vi "Dashboard Main.vi"() -> ()   [LabVIEW 2018]
uses:
  <vilib>/Utility/miscctls.llb/LVRowAndColumnTypeDef.ctl
  <vilib>/event_ctls.llb/eventvkey.ctl
  <vilib>/Rock Robotics/Network Tables/NT Read Boolean Array.vi
  <vilib>/Rock Robotics/Network Tables/NT Read Numeric Array.vi
  <vilib>/Rock Robotics/Network Tables/NT Write Numeric Array.vi
  <vilib>/Rock Robotics/Network Tables/NT Write String Array.vi
  <vilib>/Rock Robotics/WPI/Dashboard/WPI_DashboardLogging Global.vi
panel:
  in  "Camera Name":string(combo)="No Camera Selection"
  in  "Camera Settings Right":T1={"Frame Rate"=30, "Compression"=30, "Size"=1, "DB Camera Config"=FALSE} {"Frame Rate" scale=1.0..30.0; "Compression" scale=100.0..-1.0; "Size" items=["640x480", "320x240", "160x120"]}
  in  "Camera Name Right":string(combo)="No Camera Selection"
  out "Camera Perf":string
  in  "Camera Settings":T1={"Frame Rate"=30, "Compression"=30, "Size"=1, "DB Camera Config"=FALSE} {"Frame Rate" scale=1.0..30.0; "Compression" scale=100.0..-1.0; "Size" items=["640x480", "320x240", "160x120"]}
  in  "TCP":refnum<k5>
  in  "Rec Mode":enum32{"Stop", "Record", "Playback"}(radio)
  out "Robot IP":string
  out "Image Message":string="Timeout in Camera Communications"
  in  "Dashboard Tab":T2(tab)
  out "Error Message:":string
  in  "Run Automated:":bool
  out "NT Connection":bool
  out "Mode":T3(ring)=enum."Auto Disabled"
  out "Right Camera Perf":cluster{"Bandwidth (Mbps)":dbl, "FPS":dbl}
  out "Front Left Setpoint:":dbl(knob)
  out "Front Right Setpoint:":dbl(knob)
  out "Back Left Setpoint:":dbl(knob)
  out "Back Right Setpoint:":dbl(knob)
  out "Reversed Modules":bool[](array[boolean])
  in  "Write Swerve Offsets:":bool
  in  "Task:":string(combo)
  out "PositionIndicator":bool
  out "TaskIndicator":bool
  in  "Start Position:":string(combo)
  out "Camera Image Right":T4(plugin-control)
  in  "CheckList":i32(listbox)
  in  "Test Slider":dbl(slide) scale=0.0..100.0 scale format="%#_3g"
  in  "On/Off":bool caption="Solenoid"
  in  "Test Name":u16(ring) items=["Select the test to run..."]
  in  "Test Tree":string(tree)
  in  "Motor":cluster{"Value":dbl, "Enable":bool} {"Value" scale=-1.0..1.0 scale format="%#_3g"}
  out "Progress":T5 {"Test Progress" scale=0.0..100.0}
  in  "Rev/Fwd":cluster{"Forward":bool, "Reverse":bool}
  in  "Test Ring":u16(ring) items=["Monochrome", "Color"]
  out "Cmd Status":string
  in  "Execute Command":bool
  in  "Command Params":string[][](table)
  in  "Command Selection":i32(listbox)
  out "Tree":string(tree)
  out "Camera Image":T4(plugin-control)
  out "Background":bool
  # "HW"
  # "HW"
  # "Swerve Modules:"
  # "Sandstorm Options:"
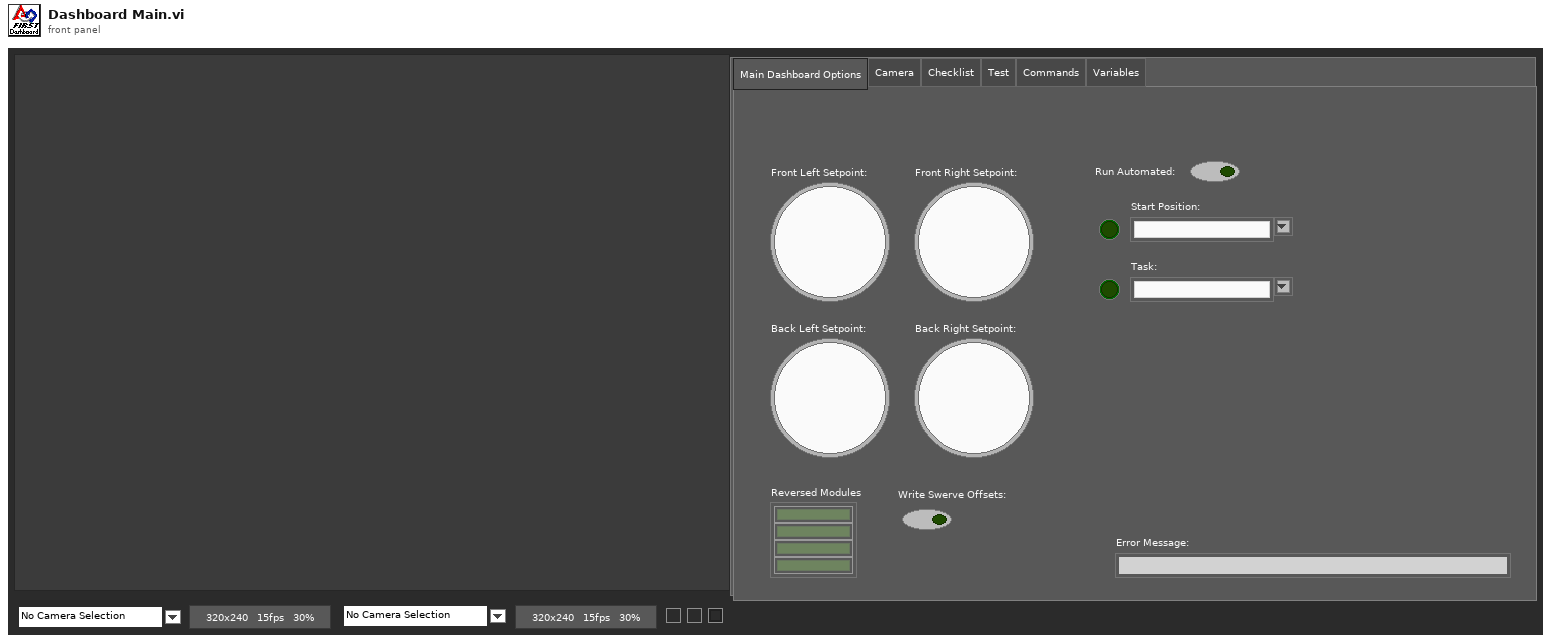
[diagram p1: front panel]
types:
  T1 = cluster{"Frame Rate":i32, "Compression":i32, "Size":u16, "DB Camera Config":bool}
  T2 = enum32{"Main Dashboard Options", "Camera", "Checklist", "Test", "Commands", "Variables"}
  T3 = enum8{"Tele-Op Disabled", "Tele-Op Enabled", "Auto Disabled", "Auto Enabled", "Test Disabled", "Test Enabled", "Disconnected", "No Code", "E-Stop"}
  T4 = typedef "IMAQ Image.ctl" = refnum<image>
  T5 = cluster{"Test Progress":u8, "Test Progress Text":string}
  T6 = cluster{"Save Path":path, "Interval (s)":dbl, "Keep":i32}
  T7 = enum32{"Drive", "Camera", "Basic", "Custom", "Test", "Commands", "Checklist", "Variables"}
  T8 = typedef "Image Type" = u32
  T9 = cluster{"IDs":cluster{"RPC field ID":u16, "Unique ID":u16}, "String":string}
  T10 = enum16{"open", "replace", "create", "open or create", "replace or create", "replace or create with confirmation"}
  T11 = cluster{"Error Strings":string, "Disable Counts":cluster{u16, u16}, "Rail Faults":cluster{u16, u16, u16}, "Robot IP":string, "DB Mode":u8, "Event Info":cluster{"Name":string, "Type":u8, "Number":u16, "Replay":u8}}
  T12 = cluster{"Storage":cluster{"Disk Free":u64, "RAM Block":u32, "RAM free":u32}, "CPU Utilization":cluster{"CPU % ISR":sgl, "CPU % Time Crit":sgl, "CPU % Timed Str":sgl, "CPU % High":sgl, "CPU % Above":sgl, "CPU % Normal":sgl, "CPU % Low":sgl}, "CAN":cluster{"% Bus Utilization":sgl, "Bus Off Cnt":u32, "TX_FIFO Full Cnt":u32, "Receive Error Cnt":u8, "Transmit Error Cnt":u8}, "HID":cluster{"HID Outputs":u32, "Rumble Low":u16, "Rumble High":u16}[]}
  T13 = cluster{"Status bits":cluster{"Test Mode":bool, "Autonomous":bool, "Enabled":bool, "Code Start":bool, "Brownout":bool, "Reserved 2":bool, "Reserved 3":bool, "E-Stop":bool}, "Code Trace":cluster{"Disabled":bool, "TeleOp":bool, "Auto":bool, "Test":bool}, "Controller Type":enum16{"unknown", "cRIO", "roboRio"}, "Code?":enum16{"unknown", "noCode", "code"}, "Battery V":dbl}
  T14 = cluster{"Control Bits":cluster{"TestMode":bool, "Autonomous":bool, "Enabled":bool, "FMS Present":bool, bool, bool, bool, "E-Stop":bool}, "Team Station ":u8, "Countdown":sgl, "Joystick Values":cluster{"Axes":dbl[], "Buttons":bool[], "POVs":i16[]}[]}
  T15 = cluster{"Camera Image":refnum<vi>, "Dashboard Tab":refnum<vi>, "Background":refnum<vi>, "Rec Mode":refnum<vi>, "Test Slider":refnum<vi>, "On/Off ":refnum<vi>, "Test Ring":refnum<vi>, "Rev/Fwd":refnum<vi>, "Test Name":refnum<vi>, "Motor":refnum<vi>, "Progress":refnum<vi>, "CheckList":refnum<vi>, "Tree":refnum<vi>, "Test Tree":refnum<vi>, "Command Params":refnum<vi>, "Command Selection":refnum<vi>, "Execute Command":refnum<vi>, "Cmd Status":refnum<vi>, "Camera Settings":refnum<vi>, "Camera Name":refnum<vi>, "Camera Perf":refnum<vi>, "Camera Settings Right":refnum<vi>, "Camera Name Right":refnum<vi>, "Camera Image Right":refnum<vi>}
  T16 = cluster{"Global Rectangle":i32[], "Contours":cluster{"Contour Type":u32, "ROI Type":u32, "Points":i32[]}[]}
  T17 = cluster{"Camera Name":string, string, "Saved DB Images Info":cluster{"Save Path":path, "Interval (s)":dbl, "Keep":i32}}
  T18 = cluster{"Camera Name Right":string, string, "Saved DB Images Info":cluster{"Save Path":path, "Interval (s)":dbl, "Keep":i32}}
  T19 = cluster{"Operation":enum16{"Update", "Clear"}, "Color Box":u32}[]
  T20 = typedef "eventvkey.ctl" = enum16{"ASCII", "Enter", "Return", "Shift", "Ctrl", "Alt", "Cmd", "Opt", "Caps", "NumLock", "Clear", "Break", "Up", "Down", "Left", "Right", "Insert", "Delete", "Home", "End", "PageUp", "PageDown", "Escape", "Help", "Pause", "ScrollLock", "F1", "F2", "F3", "F4", "F5", "F6", "F7", "F8", "F9", "F10", "F11", "F12", "F13", "F14", "F15", "F16", "F17", "F18", "F19", "F20", "F21", "F22", "F23", "F24", "Play", "VolumeUp", "VolumeDown", "Mute", "Two Byte Char"}
  T21 = cluster{"Image Size":bool, "Image Type":bool, "Pixel Value":bool, "ROI Information":bool, "Zoom Factor":bool}
  T22 = cluster{"Operation":enum16{"Update", "Clear"}, "Color Box":u32}
  T23 = typedef "LVRowAndColumnTypeDef.ctl" = cluster{"Row":i32, "Column":i32}
  T24 = cluster{"Shift":bool, "Ctrl":bool, "Alt":bool, "Cmd":bool, "Opt":bool}
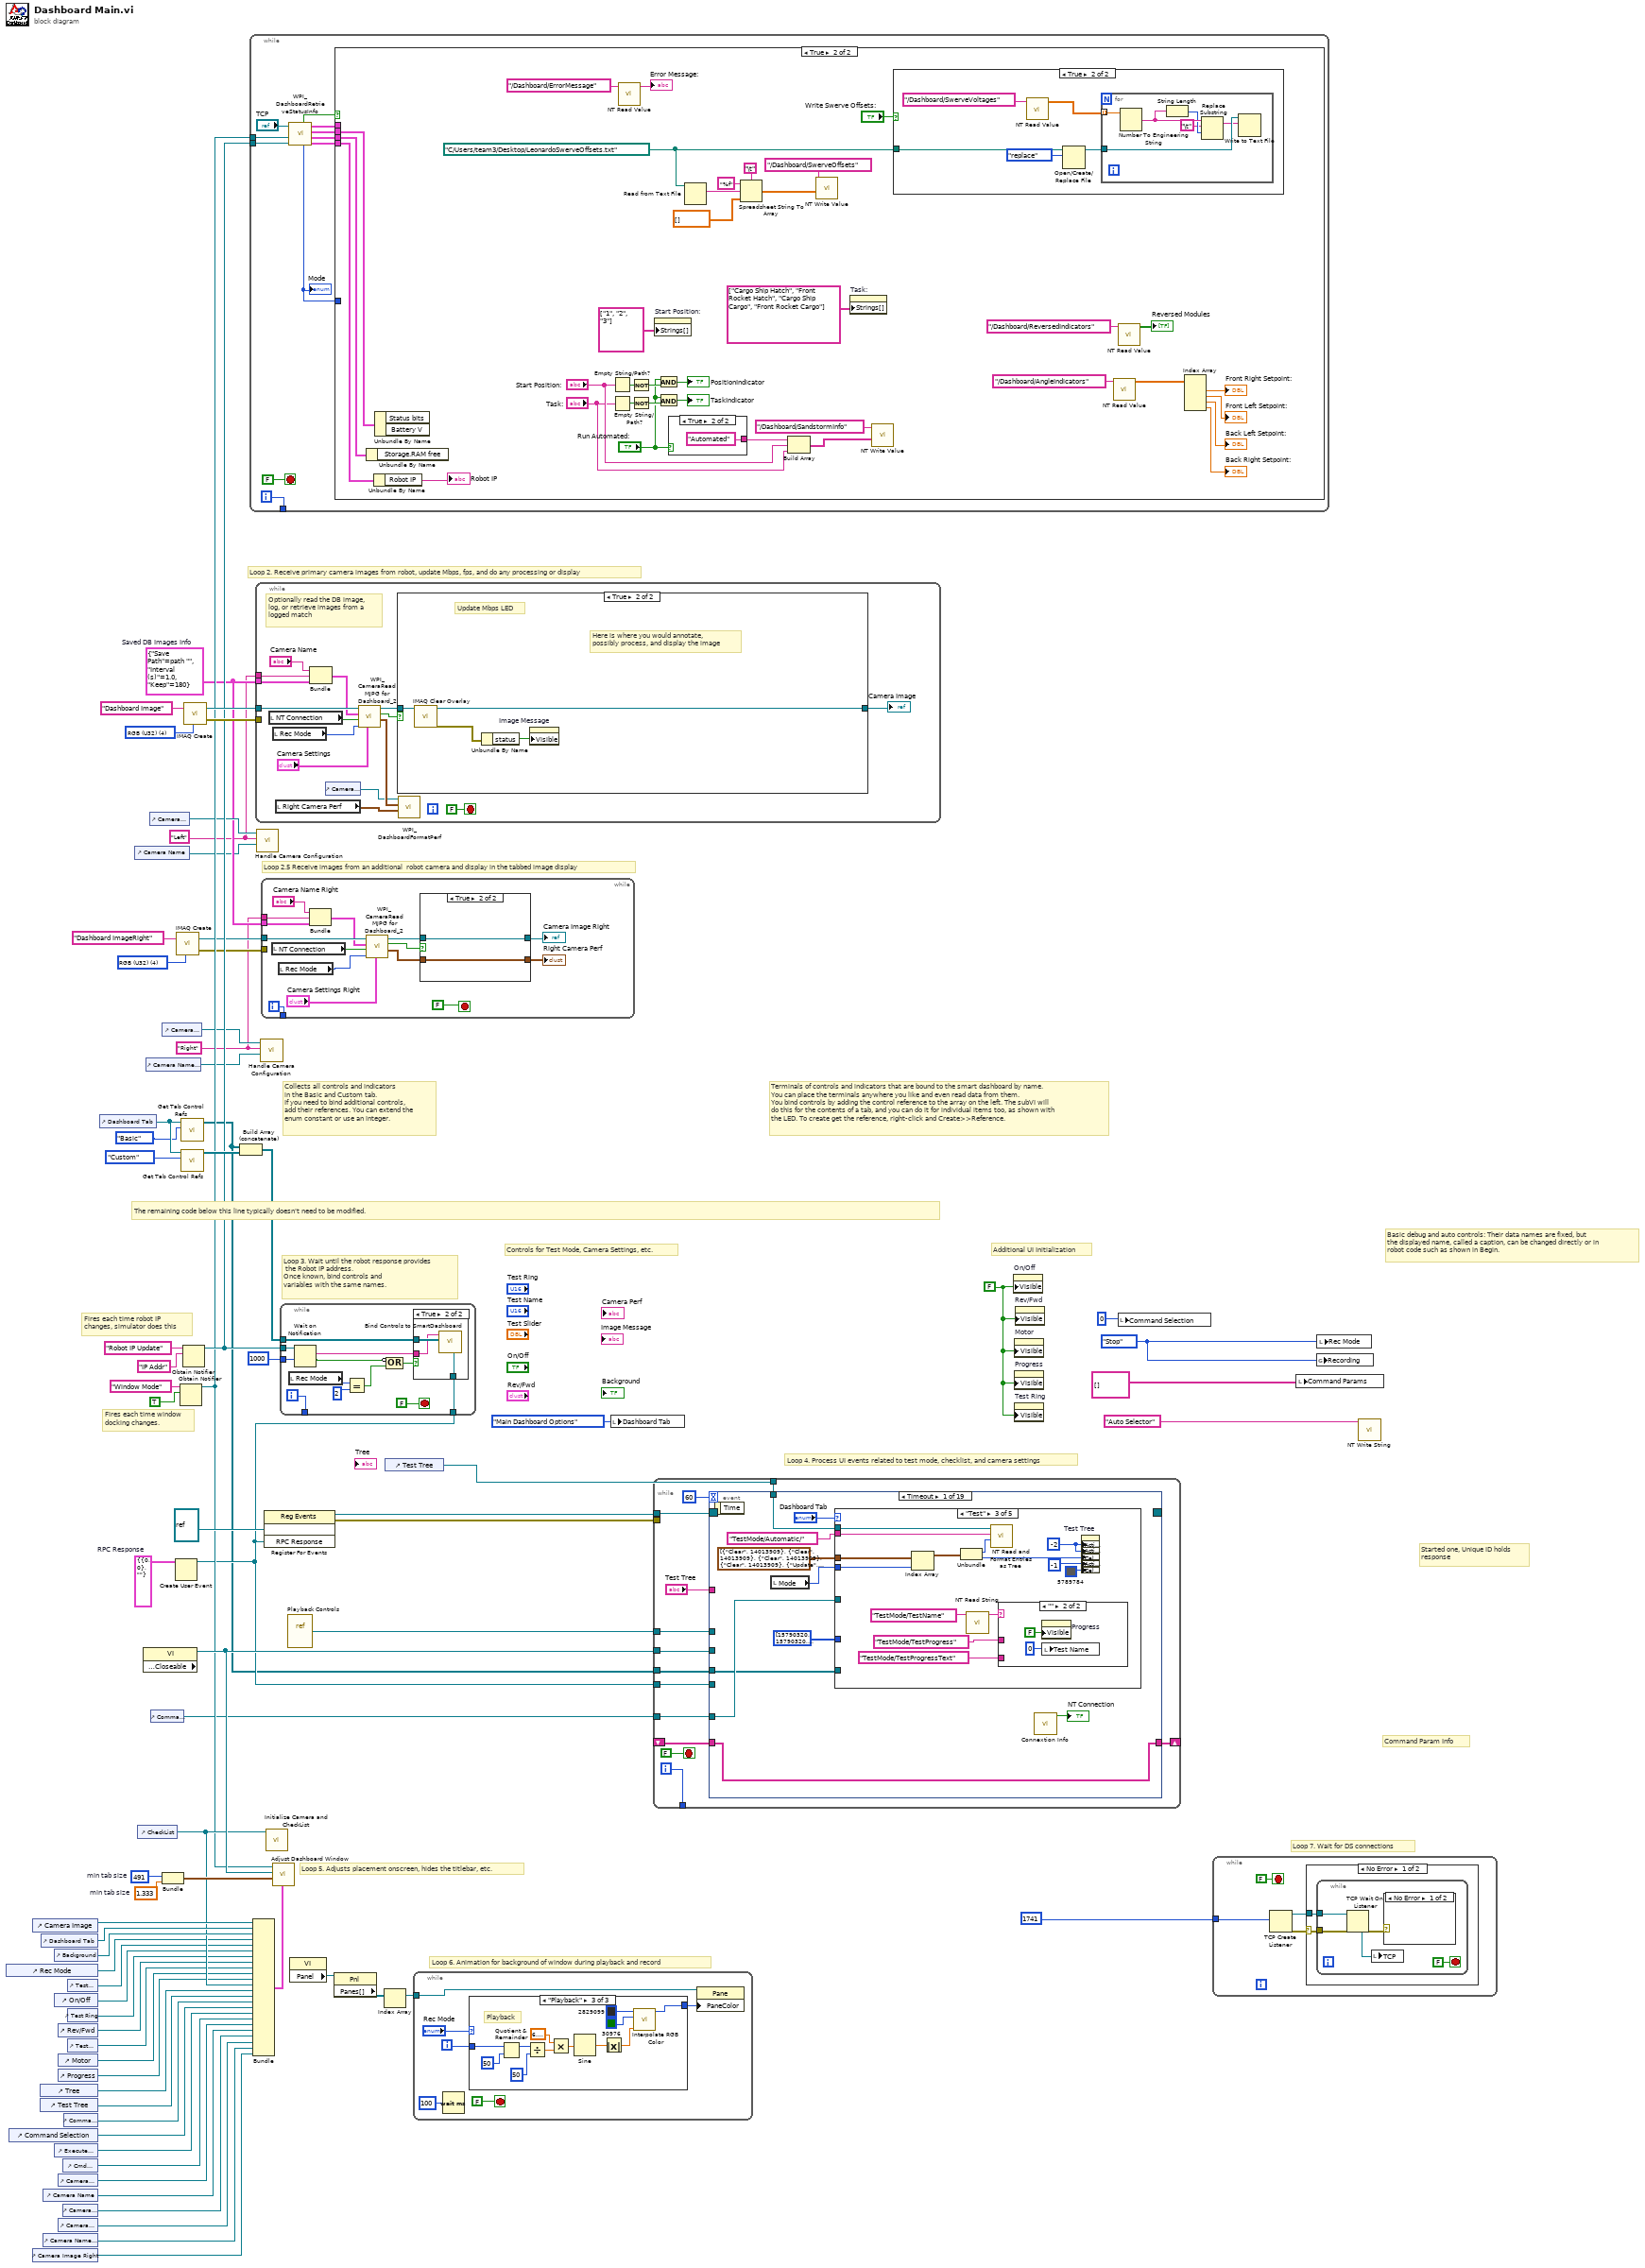
[diagram p0: block diagram]
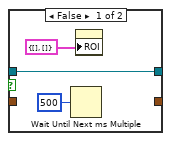
[diagram p2: hidden frame]
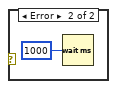
[diagram p3: hidden frame]
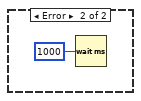
[diagram p4: hidden frame]
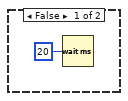
[diagram p5: hidden frame]
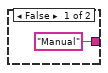
[diagram p6: hidden frame]
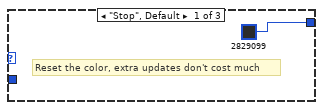
[diagram p8: hidden frame]
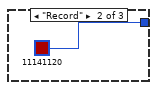
[diagram p9: hidden frame]
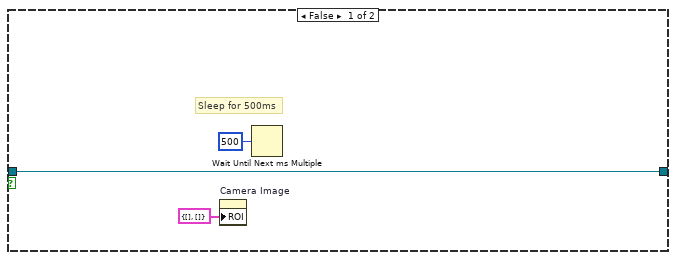
[diagram p11: hidden frame]
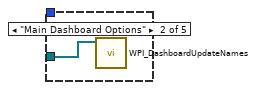
[diagram p13: hidden frame]
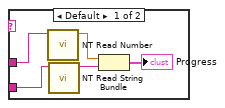
[diagram p14: hidden frame]
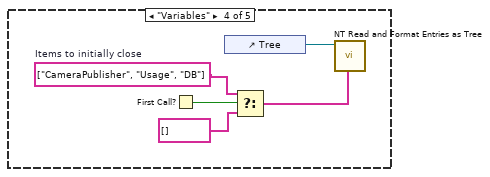
[diagram p15: hidden frame]
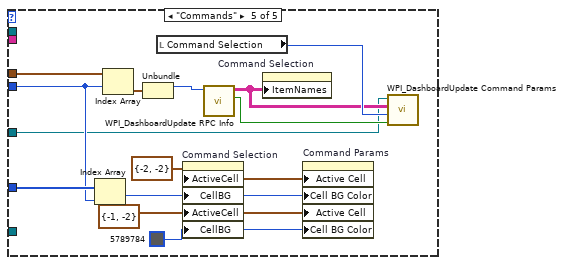
[diagram p16: hidden frame]
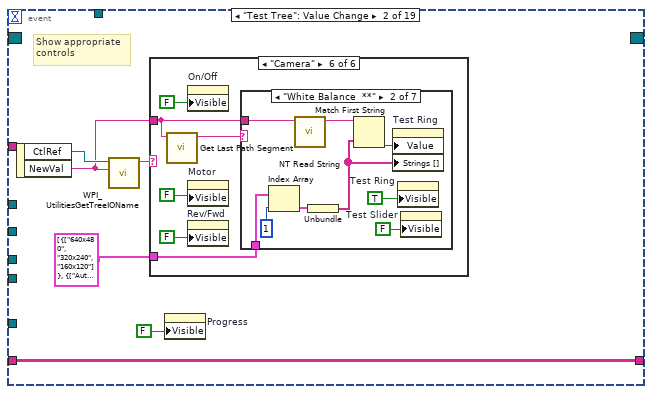
[diagram p17: hidden frame]
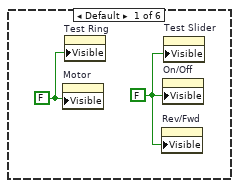
[diagram p18: hidden frame]
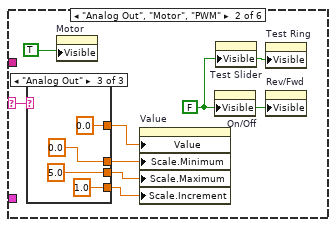
[diagram p19: hidden frame]
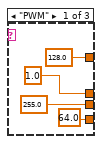
[diagram p20: hidden frame]
diagram:
  w6 = T6 {"Save Path"=path "", "Interval (s)"=1.0, "Keep"=180}  # Saved DB Images Info
  w5 = "Right"
  w4 = "Left"
  w16 = T8 4 items=["Grayscale (U8)", "Grayscale (I16)", "Grayscale (SGL)", "Complex (CSG)", "RGB (U32)", "HSL (U32)", "RGB (U64)"] ("Image Type")
  w29 = T9 {"IDs"={"RPC field ID"=0, "Unique ID"=0}, "String"=""}  # RPC Response
  w51 = 491  # min tab size
  w50 = 1.333  # min tab size
  w58 = enum32{"Stop", "Record", "Playback"}."Stop" ("Rec Mode")
  w35 = FALSE ("Visible")
  w75 = T8 4 items=["Grayscale (U8)", "Grayscale (I16)", "Grayscale (SGL)", "Complex (CSG)", "RGB (U32)", "HSL (U32)", "RGB (U64)"] ("Image Type")
  # "Loop 2.5 Receive images from an additional  robot camera and display in the tabbed image display"
  # "Command Param Info"
  # "Started one, Unique ID holds\nresponse"
  # "Loop 7. Wait for DS connections"
  # "Basic debug and auto controls: Their data names are fixed, but\nthe displayed name, called a caption, can be changed directly or in\nrobot code such as shown in Begin."
  # "Controls for Test Mode, Camera Settings, etc."
  # "Additional UI Initialization"
  # "Loop 6. Animation for background of window during playback and record"
  # "Fires each time robot IP\nchanges, simulator does this"
  # "Fires each time window\ndocking changes."
  # "Collects all controls and indicators\nin the Basic and Custom tab.\nIf you need to bind additional controls,\nadd their references. You can extend the\nenum constant or use an integer."
  # "The remaining code below this line typically doesn't need to be modified."
  # "Loop 4. Process UI events related to test mode, checklist, and camera settings"
  # "Terminals of controls and indicators that are bound to the smart dashboard by name.\nYou can place the terminals anywhere you like and even read data from them.\nYou bind controls by adding the control reference to the array on the left. The subVI will\ndo this for the contents of a tab, and you can do it for individual items too, as shown with\nthe LED. To create get the reference, right-click and Create>>Reference."
  # "Loop 3. Wait until the robot response provides\n the Robot IP address.\nOnce known, bind controls and\nvariables with the same names."
  # "Loop 5. Adjusts placement onscreen, hides the titlebar, etc."
  # "Loop 2. Receive primary camera images from robot, update Mbps, fps, and do any processing or display"
  n1 = control-ref of="Rec Mode"() -> (w41:refnum<vi>)
  n2 = control-ref of="Command Selection"() -> (w28:refnum<vi>)
  n3 = control-ref of="Camera Image"() -> (w53:refnum<vi>)
  n4 = control-ref of="Camera Image Right"() -> (w9:refnum<vi>)
  n5 = control-ref of="Tree"() -> (w45:refnum<vi>)
  n6 = control-ref of="Test Tree"() -> (w44:refnum<vi>)
  n7 = control-ref of="Dashboard Tab"() -> (w52:refnum<vi>)
  n8 = control-ref of="Camera Name"() -> (w2:refnum<vi>)
  n9 = control-ref of="Camera Name Right"() -> (w10:refnum<vi>)
  n10 = control-ref of="Background"() -> (w48:refnum<vi>)
  n11 = control-ref of="On/Off"() -> (w39:refnum<vi>)
  n12 = control-ref of="Execute Command"() -> (w30:refnum<vi>)
  n13 = control-ref of="Rev/Fwd"() -> (w37:refnum<vi>)
  n14 = control-ref of="Motor"() -> (w42:refnum<vi>)
  n15 = control-ref of="Progress"() -> (w36:refnum<vi>)
  n16 = control-ref of="Camera Settings"() -> (w21:refnum<vi>)
  n17 = control-ref of="Camera Settings Right"() -> (w11:refnum<vi>)
  n18 = control-ref of="Cmd Status"() -> (w24:refnum<vi>)
  n19 = control-ref of="Camera Perf"() -> (w20:refnum<vi>)
  n20 = control-ref of="Command Params"() -> (w31:refnum<vi>)
  n21 = control-ref of="Test Slider"() -> (w40:refnum<vi>)
  n22 = control-ref of="Test Ring"() -> (w38:refnum<vi>)
  n23 = control-ref of="Test Name"() -> (w43:refnum<vi>)
  n24 = control-ref of="Dashboard Tab"() -> (w56:refnum<vi>)
  n25 = control-ref of="Camera Name"() -> (w3:refnum<vi>)
  n26 = control-ref of="CheckList"() -> (w46:refnum<vi>)
  n27 = property class="VI" props=["Front Panel.Closeable"]() -> (reference out=w57:refnum<vi>)  [unwired: 2 in, 2 out]
  n28 = control-ref of="Camera Name Right"() -> (w12:refnum<vi>)
  n29 = control-ref of="Camera Settings"() -> (w22:refnum<vi>)
  n30 = control-ref of="Command Params"() -> (w23:refnum<vi>)
  n31 = control-ref of="Camera Settings Right"() -> (w13:refnum<vi>)
  n32 = Bundle("min tab size"=w51, "min tab size"=w50) -> (w49:cluster{"min tab size":i32, "min tab size":dbl})  [unwired: 1 in]
  n33 = Create User Event(user event datatype=w29) -> (user event=w25:refnum<user-event>)  [unwired: 1 in, 1 out]
  n34 = call "IMAQ Create"("Image Name"="Dashboard ImageRight", "Image Type"=w16) -> ("New Image"=w15:T4, "error out"=w14:errorcluster)  [unwired: 2 in, 1 out]
  n35 = Obtain Notifier(name (unnamed)="Window Mode", notification data type=TRUE) -> (notifier out=w33:refnum<notifier>)  [unwired: 2 in, 2 out]
  n36 = call <vilib>:"Get Tab Control Refs.vi"("Page Index"=T7."Basic" ("Dashboard Tab"), "TabControl in"=w56) -> ("ControlsOnPage"=w19:refnum<vi>[])  [unwired: 9 in]
  n37 = call <vilib>:"Get Tab Control Refs.vi"("Page Index"=T7."Custom" ("Dashboard Tab"), "TabControl in"=w56) -> ("ControlsOnPage"=w55:refnum<vi>[])  [unwired: 9 in]
  n38 = Obtain Notifier(name (unnamed)="Robot IP Update", notification data type="IP Addr" ("name (unnamed)")) -> (notifier out=w34:refnum<notifier>)  [unwired: 2 in, 2 out]
  n39 = call "IMAQ Create"("Image Name"="Dashboard Image", "Image Type"=w75) -> ("New Image"=w73:T4, "error out"=w72:errorcluster)  [unwired: 2 in, 1 out]
  n40 = Build Array (concatenate)(w19, w55) -> (w54:refnum<vi>[])
  n41 = while {
    tunnel: [w85] -> _
    tunnel: w34 -> [w79]
    tunnel: w33 -> [w76]
    i -> [w85]
    stop <- FALSE stop-if-true
    n42 = call <vilib>:"WPI_DashboardRetrieveStatusInfo.vi"("Binding Refnum"=w79, "Window Mode Notifier"=w76, "TCP Cnx"="TCP") -> ("Power and Errors"=w80:T11, "Robot Metrics"=w83:T12, "Status Info"=w84:T13, "Control Info"=w81:T14, "Robot Mode"=w78:T3, "Process?"=w82:bool)  [unwired: 3 in]
    "Mode" <- w78
    n43 = case shown="True" w82 {
      tunnel: w84 -> [_ w123]
      tunnel: w83 -> [_ w122]
      tunnel: w81 -> [_ _]
      tunnel: w80 -> [_ w121]
      tunnel: w78 -> [_ _]
      frame False {
        n44 = Wait (ms)(milliseconds to wait=u32 20) -> ()  [unwired: 1 out]
      }
      frame True {
        w103 = path "C:/Users/team3/Desktop/LeonardoSwerveOffsets.txt" ("file (use dialog)")
        n45 = Unbundle By Name(w122) -> ()  [unwired: 1 out]
        n46 = Unbundle By Name(w121) -> ("Robot IP"=→"Robot IP":string)
        n47 = Unbundle By Name(w123) -> ()  [unwired: 2 out]
        n48 = Empty String/Path?(string/path="Start Position:") -> (empty?=w99:bool)
        n49 = Empty String/Path?(string/path="Task:") -> (empty?=w96:bool)
        n50 = call-poly <vilib>:"NT Read Value.vi"("Name"="/Dashboard/ErrorMessage") -> ("String"=→"Error Message:":string)  [unwired: 9 in, 1 out]
        n51 = Not(x=w99) -> (.not. x?=w98:bool)
        n52 = Not(x=w96) -> (.not. x?=w97:bool)
        n53 = property on="Start Position:" class="CmbBox"("Strings[]"=string[] ["1", "2", "3"]) -> ()  [unwired: 2 in, 2 out]
        n54 = And(x="Run Automated:", y=w98) -> (x .and. y?=→"PositionIndicator":bool)
        n55 = And(x="Run Automated:", y=w97) -> (x .and. y?=→"TaskIndicator":bool)
        n56 = case shown="True" "Run Automated:" {
          tunnel: ["Manual" "Automated"] -> w93
          frame False {
          }
          frame True {
          }
        }
        n57 = Read from Text File(file (use dialog)=w103) -> (text=w117:string)  [unwired: 3 in, 3 out]
        n58 = Spreadsheet String To Array(delimiter (Tab)="\t", format string="%f", spreadsheet string=w117, array type (2D Dbl)=dbl[] []) -> (array=w116:dbl[])
        n59 = Build Array(w93, "Start Position:", "Task:") -> (w100:string[])
        n60 = call-poly <vilib>:"NT Write Value.vi"("Numeric Array"=w116, "Name"="/Dashboard/SwerveOffsets") -> ()  [unwired: 9 in, 1 out]
        n61 = property on="Task:" class="CmbBox"("Strings[]"=string[] ["Cargo Ship Hatch", "Front Rocket Hatch", "Cargo Ship Cargo", "Front Rocket Cargo"]) -> ()  [unwired: 2 in, 2 out]
        n62 = call-poly <vilib>:"NT Write Value.vi"("String Array"=w100, "Name"="/Dashboard/SandstormInfo") -> ()  [unwired: 9 in, 1 out]
        n63 = case shown="True" "Write Swerve Offsets:" {
          tunnel: w103 -> [_ w127]
          frame False {
          }
          frame True {
            n64 = call-poly <vilib>:"NT Read Value.vi"("Name"="/Dashboard/SwerveVoltages") -> ("Numeric Array"=w126:dbl[])  [unwired: 9 in, 1 out]
            n65 = Open/Create/Replace File(file path (use dialog)=w127, operation (0:open)=T10."replace") -> (refnum out=w129:refnum<file>)  [unwired: 4 in, 2 out]
            n66 = for {
              tunnel: w129 -> [w135]
              tunnel: w126 -> [w136] mode=indexing
              n67 = Number To Engineering String(4:w136) -> (0:w134:string)  [unwired: 3 in]
              n68 = String Length(string=w134) -> (length=w133:i32)
              n69 = Replace Substring(3:w133, 4:"\t", 5:w134) -> (1:w131:string)  [unwired: 1 in, 1 out]
              n70 = Write to Text File(file (use dialog)=w135, text=w131) -> ()  [unwired: 2 in, 3 out]
            }
          }
        }
        n71 = call-poly <vilib>:"NT Read Value.vi"("Name"="/Dashboard/AngleIndicators") -> ("Numeric Array"=w108:dbl[])  [unwired: 9 in, 1 out]
        n72 = call-poly <vilib>:"NT Read Value.vi"("Name"="/Dashboard/ReversedIndicators") -> ("Boolean Array"=→"Reversed Modules":bool[])  [unwired: 9 in, 1 out]
        n73 = Index Array(array=w108) -> (element #1=→"Front Right Setpoint:":dbl, element #2=→"Front Left Setpoint:":dbl, element #3=→"Back Left Setpoint:":dbl, element #4=→"Back Right Setpoint:":dbl)  [unwired: 4 in]
      }
    }
  }
  n74 = Bundle("Camera Image"=w53, "Dashboard Tab"=w52, "Background"=w48, "Rec Mode"=w41, "Test Slider"=w40, "On/Off"=w39, "Test Ring"=w38, "Rev/Fwd"=w37, "Test Name"=w43, "Motor"=w42, "Progress"=w36, "CheckList"=w46, "Tree"=w45, "Test Tree"=w44, "Command Params"=w31, "Command Selection"=w28, "Execute Command"=w30, "Cmd Status"=w24, "Camera Settings"=w21, "Camera Name"=w2, "Camera Perf"=w20, "Camera Settings Right"=w11, "Camera Name Right"=w10, "Camera Image Right"=w9) -> (w47:T15)  [unwired: 1 in]
  n75 = while {
    tunnel: w73 -> [w150]
    tunnel: w72 -> [_]
    tunnel: w6 -> [w143]
    tunnel: w4 -> [w141]
    stop <- FALSE stop-if-true
    # "Optionally read the DB image,\nlog, or retrieve images from a\nlogged match"
    n76 = local read "NT Connection"() -> (w144:bool)
    n77 = local read "Rec Mode"() -> (w147:enum32{"Stop", "Record", "Playback"})
    n78 = local read "Right Camera Perf"() -> (w139:cluster{"Bandwidth (Mbps)":dbl, "FPS":dbl})
    n79 = Bundle("Camera Name"="Camera Name", w141, "Saved DB Images Info"=w143) -> (w142:T17)  [unwired: 1 in]
    n80 = control-ref of="Camera Perf"() -> (w138:refnum<vi>)
    n81 = call <vilib>:"WPI_CameraRead MJPG for Dashboard_2.vi"("Camera Settings"="Camera Settings", "Rec Mode"=w147, "NT Connection"=w144, "Capture Info"=w142, "Image in"=w150) -> ("perf info"=w140:cluster{"Bandwidth (Mbps)":dbl, "fps":dbl}, "Active"=w148:bool, "Image\\ out"=w149:T4)  [unwired: 4 in]
    n82 = case shown="True" w148 {
      tunnel: w149 -> [w153 w156]
      tunnel: [w153 w155] -> w145
      frame False {
        # "Sleep for 500ms"
        n83 = property on="Camera Image" class="ImageControl"("ROI"=T16 {"Global Rectangle"=[], "Contours"=[]}) -> ()  [unwired: 2 in, 2 out]
        n84 = Wait Until Next ms Multiple(millisecond multiple=u32 500) -> ()  [unwired: 1 out]
      }
      frame True {
        # "Here is where you would annotate,\npossibly process, and display the image"
        # "Update Mbps LED"
        n85 = call "IMAQ Clear Overlay"("Image"=w156) -> ("error out"=w157:errorcluster, "Image Out"=w155:T4)  [unwired: 2 in, 7 out]
        n86 = Unbundle By Name(w157) -> ("status"=w158:bool)
        n87 = property on="Image Message" class="Str"("Visible"=w158) -> ()  [unwired: 2 in, 2 out]
      }
    }
    "Camera Image" <- w145
    n88 = call <vilib>:"WPI_DashboardFormatPerf.vi"("Right Camera Perf"=w139, "Performance"=w140, "String in"=w138) -> ()  [unwired: 9 in]
  }
  n89 = call "Handle Camera Configuration.vi"("CameraNameRef"=w3, "Display Name"=w4, "ClusterRef"=w22) -> ()  [unwired: 9 in]
  n90 = call "Handle Camera Configuration.vi"("CameraNameRef"=w12, "Display Name"=w5, "ClusterRef"=w13) -> ()  [unwired: 9 in]
  n91 = while {
    tunnel: w15 -> [w173]
    tunnel: w14 -> [_]
    tunnel: [w168] -> _
    tunnel: w6 -> [w164]
    tunnel: w5 -> [w161]
    i -> [w168]
    stop <- FALSE stop-if-true
    n92 = local read "NT Connection"() -> (w165:bool)
    n93 = local read "Rec Mode"() -> (w172:enum32{"Stop", "Record", "Playback"})
    n94 = Bundle("Camera Name Right"="Camera Name Right", w161, "Saved DB Images Info"=w164) -> (w163:T18)  [unwired: 1 in]
    n95 = call <vilib>:"WPI_CameraRead MJPG for Dashboard_2.vi"("Camera Settings"="Camera Settings Right", "Rec Mode"=w172, "NT Connection"=w165, "Capture Info"=w163, "Image in"=w173) -> ("perf info"=w159:cluster{"Bandwidth (Mbps)":dbl, "fps":dbl}, "Active"=w167:bool, "Image\\ out"=w170:T4)  [unwired: 4 in]
    n96 = case shown="True" w167 {
      tunnel: w170 -> [w175 w178]
      tunnel: [w175 w178] -> w166
      tunnel: [_ w177] -> w160
      tunnel: w159 -> [_ w177]
      frame False {
        n97 = Wait Until Next ms Multiple(millisecond multiple=u32 500) -> ()  [unwired: 1 out]
        n98 = property on="Camera Image Right" class="ImageControl"("ROI"=T16 {"Global Rectangle"=[], "Contours"=[]}) -> ()  [unwired: 2 in, 2 out]
      }
      frame True {
      }
    }
    "Camera Image Right" <- w166
    "Right Camera Perf" <- w160
  }
  n99 = register-events(refnum<vi> refnum, w25) -> (reference out=w62:refnum<event-registration>, error out=w61:errorcluster)  [unwired: 2 in]
  n100 = call "Initialize Camera and CheckList.vi"("ListBox in"=w46) -> ()  [unwired: 11 in]
  n101 = call "Adjust Dashboard Window.vi"("Sizing Refnums"=w47, "Size Constraints"=w49, "VI"=w57, "WIn Mode"=w33) -> ()  [unwired: 8 in]
  n102 = while {
    tunnel: w54 -> [w190]
    tunnel: w34 -> [w188]
    tunnel: [w186] -> _
    tunnel: u32 1000 ("milliseconds to wait") -> [w185]
    tunnel: w25 -> [w179]
    i -> [w186]
    stop <- FALSE stop-if-true
    n103 = local read "Rec Mode"() -> (w181:enum32{"Stop", "Record", "Playback"})
    n104 = Wait on Notification(notifier=w188, timeout in ms (-1)=w185) -> (notification=w187:string, timed out?=w183:bool)  [unwired: 2 in, 2 out]
    n105 = Equal?(x=w181, y=u16 2 ("Rec Mode")) -> (x = y?=w182:bool)
    n106 = Compound Arithmetic op=OR(invert w183, w182) -> (w184:bool)
    n107 = case shown="True" w184 {
      tunnel: w190 -> [_ w193]
      tunnel: w187 -> [_ w192]
      tunnel: w179 -> [_ w191]
      frame False {
      }
      frame True {
        n108 = call <vilib>:"Bind Controls to SmartDashboard.vi"("RPC ref"=w191, "Bound Control Refs"=w193, "Server IP Address"=w192) -> ()  [unwired: 9 in]
      }
    }
  }
  n109 = vi-ref "Playback Controls.vi"() -> (w63:refnum<vi>)
  n110 = property class="VI"() -> ("Panel"=w65:refnum<vi>)  [unwired: 2 in, 2 out]
  n111 = property class="Pnl"(reference=w65) -> ("Panes[]"=w66:refnum<vi>[])  [unwired: 1 in, 2 out]
  n112 = Index Array(array=w66) -> (element=w64:refnum<vi>)  [unwired: 1 in]
  n113 = control-ref of="Test Tree"() -> (w67:refnum<vi>)
  n114 = while {
    tunnel: w64 -> [w195]
    i -> [w198]
    stop <- FALSE stop-if-true
    n115 = Wait (ms)(milliseconds to wait=u32 100) -> ()  [unwired: 1 out]
    n116 = case shown="\"Playback\"" "Rec Mode" {
      tunnel: w198 -> [_ _ w213]
      tunnel: [u32 2829099 ("Base Color") u32 11141120 ("Target Color") w202] -> w194
      frame "Stop", Default {
        # "Reset the color, extra updates don't cost much"
      }
      frame "Record" {
      }
      frame "Playback" {
        # "Playback"
        n117 = Quotient & Remainder(x=w213, y=u32 50 ("milliseconds to wait")) -> (x-y*floor(x/y)=w209:u32)  [unwired: 1 out]
        n118 = Divide(x=w209, y=u32 50 ("milliseconds to wait")) -> (x/y=w206:dbl)
        n119 = Multiply(x=6.283185307179586, y=w206) -> (x*y=w211:dbl)
        n120 = Sine(x=w211) -> (sin(x)=w210:dbl)
        n121 = Absolute Value(x=w210) -> (abs(x)=w203:dbl)
        n122 = call "Interpolate RGB Color.vi"("Proportion"=w203, "Target Color"=u32 30976, "Base Color"=u32 2829099) -> ("Result Color"=w202:u32)  [unwired: 8 in]
      }
    }
    n123 = property class="Pane"(reference=w195, "PaneColor"=w194) -> ()  [unwired: 1 in, 2 out]
  }
  n124 = local write "Dashboard Tab"(T2."Main Dashboard Options" ("Dashboard Tab")) -> ()
  n125 = while {
    tunnel: [w223] -> _
    tunnel: w67 -> [w222]
    tunnel: w63 -> [w221]
    tunnel: w62 -> [w220]
    tunnel: w61 -> [_]
    tunnel: w57 -> [w219]
    tunnel: w25 -> [w218]
    tunnel: w23 -> [w217]
    shift-right: [w216] -> _
    shift-left: _ -> [w215]
    tunnel: w19 -> [w214]
    i -> [w223]
    stop <- FALSE stop-if-true
    n126 = event shown="[0] Timeout" {
      selector: w220 -> [_ _ _ _ _ _ _ _ _ _ _ _ _ _ _ _ _ _ _]
      dyn-events: [_ _ _ _ _ _ _ _ _ _ _ _ _ _ w477 _ _ _ _] -> _
      timeout: u32 60 ("milliseconds to wait") -> [_ _ _ _ _ _ _ _ _ _ _ _ _ _ _ _ _ _ _]
      tunnel: w222 -> [w235 _ _ _ _ _ _ _ _ _ _ _ _ _ _ _ _ _ _]
      tunnel: "Test Tree" -> [_ _ _ _ _ _ _ _ _ w444 w452 w454 w458 w466 _ _ _ _ _]
      tunnel: w221 -> [_ _ _ _ _ _ _ _ _ _ _ _ _ _ w479 _ w497 _ _]
      tunnel: w219 -> [_ _ _ _ _ _ _ _ _ _ _ _ _ _ w475 _ _ _ _]
      tunnel: w218 -> [_ _ _ _ _ _ _ _ _ _ _ _ _ _ w473 _ _ _ _]
      tunnel: w217 -> [w230 _ _ _ w395 _ _ _ _ _ _ _ _ _ _ _ _ _ _]
      tunnel: [w229 w278 w380 w385 w393 w402 w412 w419 w431 w443 w450 w453 w457 w465 w472 w492 w494 w498 w511] -> w216
      tunnel: w215 -> [w229 w278 w380 w385 w393 _ _ w419 w431 w443 w450 w453 w457 w465 w472 w492 w494 w498 w511]
      tunnel: w214 -> [w227 _ _ _ _ _ _ _ _ _ _ _ _ _ _ _ _ _ _]
      event Timeout {
        n127 = event-data() -> ()  [unwired: 1 in, 1 out]
        n128 = local read "Mode"() -> (w232:T3)
        n129 = case shown="\"Test\"" "Dashboard Tab" {
          tunnel: w235 -> [_ _ w251 _ _]
          tunnel: "TestMode/Automatic/" ("Name Pattern") -> [_ _ w250 _ _]
          tunnel: T19 [{"Operation"=enum."Clear", "Color Box"=14013909}, {"Operation"=enum."Clear", "Color Box"=14013909}, {"Operation"=enum."Clear", "Color Box"=14013909}, {"Operation"=enum."Clear", "Color Box"=14013909}, {"Operation"=enum."Update", "Color Box"=14013909}, {"Operation"=enum."Update", "Color Box"=16777215}, {"Operation"=enum."Clear", "Color Box"=14013909}, {"Operation"=enum."Clear", "Color Box"=14013909}, {"Operation"=enum."Clear", "Color Box"=14013909}] -> [_ _ w243 _ w271]
          tunnel: w232 -> [_ _ w242 _ w270]
          tunnel: u32[] [15790320, 15790320, 15790320, 15790320, 16777215, 16777215, 15790320, 15790320, 15790320] -> [_ _ _ _ w276]
          tunnel: w230 -> [_ _ _ _ w264]
          tunnel: w227 -> [_ w237 _ _ _]
          frame "Camera", Default {
          }
          frame "Main Dashboard Options" {
            n130 = call <vilib>:"WPI_DashboardUpdateNames.vi"("Controls on Tab"=w237) -> ()  [unwired: 11 in]
          }
          frame "Test" {
            w249 = -2 ("Active Item:Row Number")
            n131 = Index Array(array=w243, index=w242) -> (element=w244:T22)
            n132 = Unbundle(w244) -> ("Operation"=w245:enum16{"Update", "Clear"}, "Color Box"=w246:u32)
            n133 = call <vilib>:"NT Read String.vi"("Name"="TestMode/TestName") -> ("String"=w240:string)  [unwired: 9 in, 1 out]
            n134 = call <vilib>:"NT Read and Format Entries as Tree.vi"("Operation"=w245, "Name Pattern"=w250, "Tree Refnum"=w251) -> ()  [unwired: 7 in, 2 out]
            n135 = case shown="\"\"" w240 {
              tunnel: "TestMode/TestProgress" ("Name") -> [w253 _]
              tunnel: "TestMode/TestProgressText" ("Name") -> [w252 _]
              frame Default {
                n136 = call <vilib>:"NT Read Number.vi"("Name"=w253) -> ("Numeric"=w254:dbl)  [unwired: 9 in, 1 out]
                n137 = call <vilib>:"NT Read String.vi"("Name"=w252) -> ("String"=w255:string)  [unwired: 9 in, 1 out]
                n138 = Bundle("Numeric"=w254, "String"=w255) -> (→"Progress":cluster{"Numeric":dbl, "String":string})  [unwired: 1 in]
              }
              frame "" {
                n139 = property on="Progress" class="Clust (strict)"("Visible"=FALSE) -> ()  [unwired: 2 in, 2 out]
                n140 = local write "Test Name"(u16 0) -> ()
              }
            }
            n141 = property on="Test Tree" class="Tree (strict)"("Active Item Row Number"=w249, "ActiveColNum"=w249, "CellBG"=w246, "Active Item Row Number"=-1 ("Active Item:Row Number"), "CellBG"=u32 5789784 ("Color Box")) -> ()  [unwired: 2 in, 2 out]
          }
          frame "Variables" {
            w261 = string[] ["CameraPublisher", "Usage", "DB"]  # Items to initially close
            n142 = First Call?() -> (First Call?: T/F=w262:bool)
            n143 = control-ref of="Tree"() -> (w263:refnum<vi>)
            n144 = Select(t=w261, s=w262, f=string[] []) -> (s? t:f=w259:string[])
            n145 = call <vilib>:"NT Read and Format Entries as Tree.vi"("Tags to  Close"=w259, "Tree Refnum"=w263) -> ()  [unwired: 8 in, 2 out]
          }
          frame "Commands" {
            w272 = u32 5789784 ("Color Box")
            w273 = T23 {"Row"=-1, "Column"=-2} ("Active Cell:Active Cell")
            w275 = T23 {"Row"=-2, "Column"=-2} ("Active Cell:Active Cell")
            n146 = Index Array(array=w276, index=w270) -> (element=w274:u32)
            n147 = Index Array(array=w271, index=w270) -> (element=w269:T22)
            n148 = Unbundle(w269) -> ("Operation"=w268:enum16{"Update", "Clear"})  [unwired: 1 out]
            n149 = local read "Command Selection"() -> (w267:i32)
            n150 = property on="Command Selection" class="MCListbox (strict)"("ActiveCell"=w275, "CellBG"=w274, "ActiveCell"=w273, "CellBG"=w272) -> ()  [unwired: 2 in, 2 out]
            n151 = call <vilib>:"WPI_DashboardUpdate RPC Info.vi"("Operation"=w268) -> ("update"=w266:bool, "commands"=w265:string[][])  [unwired: 9 in]
            n152 = property on="Command Selection" class="MCListbox (strict)"("ItemNames"=w265) -> ()  [unwired: 2 in, 2 out]
            n153 = property on="Command Params" class="Tbl (strict)"("Active Cell"=w275, "Cell BG Color"=w274, "Active Cell"=w273, "Cell BG Color"=w272) -> ()  [unwired: 2 in, 2 out]
            n154 = call <vilib>:"WPI_DashboardUpdate Command Params.vi"("Update"=w266, "NewVal"=w267, "Commands"=w265, "Param Tbl"=w264) -> ()  [unwired: 7 in, 1 out]
          }
        }
        n155 = call <vilib>:"Connextion Info.vi"() -> ("Connected"=→"NT Connection":bool)  [unwired: 10 in, 1 out]
      }
      event "Test Tree": Value Change {
        # "Show appropriate\ncontrols"
        n156 = event-data() -> ("CtlRef"=w281:refnum<vi>, "NewVal"=w279:string)  [unwired: 1 in]
        n157 = call <vilib>:"WPI_UtilitiesGetTreeIOName.vi"("NewVal"=w279, "TreeControl in"=w281) -> ("I/O Name"=w282:string)  [unwired: 9 in]
        n158 = case shown="\"Camera\"" w282 {
          selector: w282 -> [_ w289 _ w311 w320 _]
          tunnel: w279 -> [_ _ w308 w310 _ w327]
          tunnel: cluster{string[]}[] [{["640x480", "320x240", "160x120"]}, {["Auto", "Fixed indoor", "Fixed outdoor 1", "Fixed outdoor 2", "Fixed fluorescent 1", "Fixed fluorescent 2", "Hold current"]}, {["Auto", "Flicker-free 50 Hz", "Flicker-free 60 Hz", "Hold current"]}, {["None", "Prioritize frame rate", "Prioritize image quality"]}, {["Monochrome", "Color"]}] -> [_ _ _ _ _ w326]
          frame Default {
            w284 = FALSE ("Visible")
            w283 = FALSE ("Visible")
            n159 = property on="Motor" class="Clust (strict)"("Visible"=w283) -> ()  [unwired: 2 in, 2 out]
            n160 = property on="Test Ring" class="Ring (strict)"("Visible"=w283) -> ()  [unwired: 2 in, 2 out]
            n161 = property on="Rev/Fwd" class="Clust (strict)"("Visible"=w284) -> ()  [unwired: 2 in, 2 out]
            n162 = property on="On/Off" class="Bool (strict)"("Visible"=w284) -> ()  [unwired: 2 in, 2 out]
            n163 = property on="Test Slider" class="Slide (strict)"("Visible"=w284) -> ()  [unwired: 2 in, 2 out]
          }
          frame "Analog Out", "Motor", "PWM" {
            w290 = FALSE ("Visible")
            n164 = case shown="\"Analog Out\"" w289 {
              tunnel: [1.0 ("Value") -1.0 ("Value") 0.0 ("Value")] -> w288
              tunnel: [255.0 ("Value") 1.0 ("Value") 5.0 ("Value")] -> w287
              tunnel: [128.0 ("Value") 0.0 ("Value") 0.0 ("Value")] -> w286
              tunnel: [64.0 ("Value") 0.5 ("Value") 1.0 ("Value")] -> w285
              frame "PWM" {
              }
              frame "Motor", Default {
              }
              frame "Analog Out" {
              }
            }
            n165 = property on="Motor" class="Clust (strict)"("Visible"=TRUE) -> ()  [unwired: 2 in, 2 out]
            n166 = property on="Value" class="Slide (strict)"("Value"=w286, "Scale.Minimum"=w288, "Scale.Maximum"=w287, "Scale.Increment"=w285) -> ()  [unwired: 2 in, 2 out]
            n167 = property on="On/Off" class="Bool (strict)"("Visible"=w290) -> ()  [unwired: 2 in, 2 out]
            n168 = property on="Test Slider" class="Slide (strict)"("Visible"=w290) -> ()  [unwired: 2 in, 2 out]
            n169 = property on="Test Ring" class="Ring (strict)"("Visible"=w290) -> ()  [unwired: 2 in, 2 out]
            n170 = property on="Rev/Fwd" class="Clust (strict)"("Visible"=w290) -> ()  [unwired: 2 in, 2 out]
          }
          frame "Servo" {
            w306 = FALSE ("Visible")
            n171 = call <vilib>:"NT Read Number.vi"("Name"=w308) -> ("Numeric"=w307:dbl)  [unwired: 9 in, 1 out]
            n172 = property on="Test Slider" class="Slide (strict)"("Visible"=TRUE, "Scale.Maximum"=170.0 ("Scale.Range:Maximum")) -> ()  [unwired: 2 in, 2 out]
            n173 = local write "Test Slider"(w307) -> ()
            n174 = property on="Motor" class="Clust (strict)"("Visible"=w306) -> ()  [unwired: 2 in, 2 out]
            n175 = property on="Rev/Fwd" class="Clust (strict)"("Visible"=w306) -> ()  [unwired: 2 in, 2 out]
            n176 = property on="On/Off" class="Bool (strict)"("Visible"=w306) -> ()  [unwired: 2 in, 2 out]
            n177 = property on="Test Ring" class="Ring (strict)"("Visible"=w306) -> ()  [unwired: 2 in, 2 out]
          }
          frame "Relay", "Solenoid" {
            w309 = FALSE ("Visible")
            n178 = property on="Motor" class="Clust (strict)"("Visible"=w309) -> ()  [unwired: 2 in, 2 out]
            n179 = property on="Test Slider" class="Slide (strict)"("Visible"=w309) -> ()  [unwired: 2 in, 2 out]
            n180 = Search and Replace String(input string=w310, search string="/Value  **", replace string="/Direction") -> (result string=w316:string)  [unwired: 5 in, 3 out]
            n181 = property on="Test Ring" class="Ring (strict)"("Visible"=w309) -> ()  [unwired: 2 in, 2 out]
            n182 = call <vilib>:"NT Read String.vi"("Name"=w316) -> ("String"=w314:string)  [unwired: 9 in, 1 out]
            n183 = Equal?(x="Both directions", y=w314) -> (x = y?=w312:bool)
            n184 = Not(x=w312) -> (.not. x?=w313:bool)
            n185 = property on="Rev/Fwd" class="Clust (strict)"("Visible"=w312) -> ()  [unwired: 2 in, 2 out]
            n186 = property on="On/Off" class="Bool (strict)"("Visible"=w313, "Caption.Text"=w311) -> ()  [unwired: 2 in, 2 out]
          }
          frame "Compressor", "Digital Out" {
            w319 = FALSE ("Visible")
            # "Get direction and finish"
            n187 = property on="Motor" class="Clust (strict)"("Visible"=w319) -> ()  [unwired: 2 in, 2 out]
            n188 = property on="Test Slider" class="Slide (strict)"("Visible"=w319) -> ()  [unwired: 2 in, 2 out]
            n189 = property on="Test Ring" class="Ring (strict)"("Visible"=w319) -> ()  [unwired: 2 in, 2 out]
            n190 = property on="On/Off" class="Bool (strict)"("Visible"=TRUE, "Caption.Text"=w320) -> ()  [unwired: 2 in, 2 out]
            n191 = property on="Rev/Fwd" class="Clust (strict)"("Visible"=FALSE) -> ()  [unwired: 2 in, 2 out]
          }
          frame "Camera" {
            n192 = call <vilib>:"Get Last Path Segment.vi"("String in"=w327) -> ("String out"=w328:string)  [unwired: 10 in]
            n193 = property on="On/Off" class="Bool (strict)"("Visible"=FALSE) -> ()  [unwired: 2 in, 2 out]
            n194 = property on="Motor" class="Clust (strict)"("Visible"=FALSE) -> ()  [unwired: 2 in, 2 out]
            n195 = property on="Rev/Fwd" class="Clust (strict)"("Visible"=FALSE) -> ()  [unwired: 2 in, 2 out]
            n196 = case shown="\"White Balance  **\"" w328 {
              tunnel: w327 -> [w334 w343 w352 w361 w370 _ w376]
              tunnel: w326 -> [w332 w340 w349 w358 w367 _ _]
              frame "Size  **" {
                n197 = Index Array(array=w332) -> (element=w331:cluster{string[]})  [unwired: 1 in]
                n198 = call <vilib>:"NT Read String.vi"("Name"=w334) -> ("String"=w333:string)  [unwired: 9 in, 1 out]
                n199 = Unbundle(w331) -> (w329:string[])
                n200 = Match First String(2:w329, 3:w333) -> (0:w330:i32)  [unwired: 1 out]
                n201 = property on="Test Ring" class="Ring (strict)"("Value"=w330, "Strings []"=w329) -> ()  [unwired: 2 in, 2 out]
                n202 = property on="Test Ring" class="Ring (strict)"("Visible"=TRUE) -> ()  [unwired: 2 in, 2 out]
                n203 = property on="Test Slider" class="Slide (strict)"("Visible"=FALSE) -> ()  [unwired: 2 in, 2 out]
              }
              frame "White Balance  **" {
                n204 = Index Array(array=w340, index=1) -> (element=w341:cluster{string[]})
                n205 = call <vilib>:"NT Read String.vi"("Name"=w343) -> ("String"=w342:string)  [unwired: 9 in, 1 out]
                n206 = Unbundle(w341) -> (w338:string[])
                n207 = Match First String(2:w338, 3:w342) -> (0:w337:i32)  [unwired: 1 out]
                n208 = property on="Test Ring" class="Ring (strict)"("Value"=w337, "Strings []"=w338) -> ()  [unwired: 2 in, 2 out]
                n209 = property on="Test Ring" class="Ring (strict)"("Visible"=TRUE) -> ()  [unwired: 2 in, 2 out]
                n210 = property on="Test Slider" class="Slide (strict)"("Visible"=FALSE) -> ()  [unwired: 2 in, 2 out]
              }
              frame "Exposure  **" {
                n211 = Index Array(array=w349, index=2) -> (element=w350:cluster{string[]})
                n212 = call <vilib>:"NT Read String.vi"("Name"=w352) -> ("String"=w351:string)  [unwired: 9 in, 1 out]
                n213 = Unbundle(w350) -> (w346:string[])
                n214 = Match First String(2:w346, 3:w351) -> (0:w347:i32)  [unwired: 1 out]
                n215 = property on="Test Ring" class="Ring (strict)"("Value"=w347, "Strings []"=w346) -> ()  [unwired: 2 in, 2 out]
                n216 = property on="Test Ring" class="Ring (strict)"("Visible"=TRUE) -> ()  [unwired: 2 in, 2 out]
                n217 = property on="Test Slider" class="Slide (strict)"("Visible"=FALSE) -> ()  [unwired: 2 in, 2 out]
              }
              frame "Exposure Priority  **" {
                n218 = Index Array(array=w358, index=3) -> (element=w359:cluster{string[]})
                n219 = call <vilib>:"NT Read String.vi"("Name"=w361) -> ("String"=w360:string)  [unwired: 9 in, 1 out]
                n220 = Unbundle(w359) -> (w355:string[])
                n221 = Match First String(2:w355, 3:w360) -> (0:w356:i32)  [unwired: 1 out]
                n222 = property on="Test Ring" class="Ring (strict)"("Value"=w356, "Strings []"=w355) -> ()  [unwired: 2 in, 2 out]
                n223 = property on="Test Ring" class="Ring (strict)"("Visible"=TRUE) -> ()  [unwired: 2 in, 2 out]
                n224 = property on="Test Slider" class="Slide (strict)"("Visible"=FALSE) -> ()  [unwired: 2 in, 2 out]
              }
              frame "Color Enable  **" {
                n225 = Index Array(array=w367, index=4) -> (element=w368:cluster{string[]})
                n226 = call <vilib>:"NT Read String.vi"("Name"=w370) -> ("String"=w369:string)  [unwired: 9 in, 1 out]
                n227 = Unbundle(w368) -> (w364:string[])
                n228 = Match First String(2:w364, 3:w369) -> (0:w365:i32)  [unwired: 1 out]
                n229 = property on="Test Ring" class="Ring (strict)"("Value"=w365, "Strings []"=w364) -> ()  [unwired: 2 in, 2 out]
                n230 = property on="Test Ring" class="Ring (strict)"("Visible"=TRUE) -> ()  [unwired: 2 in, 2 out]
                n231 = property on="Test Slider" class="Slide (strict)"("Visible"=FALSE) -> ()  [unwired: 2 in, 2 out]
              }
              frame Default {
                n232 = property on="Test Ring" class="Ring (strict)"("Visible"=FALSE) -> ()  [unwired: 2 in, 2 out]
                n233 = property on="Test Slider" class="Slide (strict)"("Visible"=FALSE) -> ()  [unwired: 2 in, 2 out]
              }
              frame "Brightness  **", "Color Level  **", "Compression  **", "FPS  **", "Sharpness  **" {
                n234 = call <vilib>:"NT Read Number.vi"("Name"=w376) -> ("Numeric"=w375:dbl)  [unwired: 9 in, 1 out]
                n235 = local write "Test Slider"(w375) -> ()
                n236 = property on="Test Slider" class="Slide (strict)"("Visible"=TRUE, "Scale.Maximum"=100.0 ("Scale.Range:Maximum")) -> ()  [unwired: 2 in, 2 out]
                n237 = property on="Test Ring" class="Ring (strict)"("Visible"=FALSE) -> ()  [unwired: 2 in, 2 out]
              }
            }
          }
        }
        n238 = property on="Progress" class="Clust (strict)"("Visible"=FALSE) -> ()  [unwired: 2 in, 2 out]
      }
      event "Test Name": Mouse Enter {
        # "Populate the ring with the list of tests"
        n239 = event-data() -> ()  [unwired: 1 in, 1 out]
        n240 = call <vilib>:"NT Read String Array.vi"("Name"="TestMode/TestList") -> ("String Array"=w384:string[])  [unwired: 9 in, 1 out]
        n241 = Build Array (concatenate)("Select the test to run...", w384) -> (w383:string[])
        n242 = property on="Test Name" class="Ring (strict)"("Strings []"=w383) -> ()  [unwired: 2 in, 2 out]
      }
      event "Test Name": Value Change {
        w386 = FALSE ("Visible")
        # "Tell the robot the test name to run"
        n243 = event-data() -> ("NewVal"=w390:u16)  [unwired: 1 in]
        n244 = property on="Test Name" class="Ring (strict)"() -> ("Strings []"=w391:string[])  [unwired: 2 in, 2 out]
        n245 = local write "Progress"(T5 {"Test Progress"=0, "Test Progress Text"=""} ("Progress")) -> ()
        n246 = Index Array(array=w391, index=w390) -> (element=w389:string)
        n247 = call <vilib>:"NT Write String.vi"("String"=w389, "Name"="TestMode/TestName") -> ()  [unwired: 9 in, 1 out]
        n248 = property on="Progress" class="Clust (strict)"("Visible"=TRUE) -> ()  [unwired: 2 in, 2 out]
        n249 = property on="Motor" class="Clust (strict)"("Visible"=w386) -> ()  [unwired: 2 in, 2 out]
        n250 = property on="Test Slider" class="Slide (strict)"("Visible"=w386) -> ()  [unwired: 2 in, 2 out]
        n251 = property on="On/Off" class="Bool (strict)"("Visible"=w386) -> ()  [unwired: 2 in, 2 out]
        n252 = property on="Rev/Fwd" class="Clust (strict)"("Visible"=w386) -> ()  [unwired: 2 in, 2 out]
        n253 = property on="Test Ring" class="Ring (strict)"("Visible"=w386) -> ()  [unwired: 2 in, 2 out]
      }
      event "Command Selection": Value Change {
        # "Get the params and show in table"
        n254 = event-data() -> ("NewVal"=w396:i32)  [unwired: 1 in]
        n255 = property on="Command Selection" class="MCListbox (strict)"() -> ("ItemNames"=w394:string[][])  [unwired: 2 in, 2 out]
        n256 = call <vilib>:"WPI_DashboardUpdate Command Params.vi"("NewVal"=w396, "Commands"=w394, "Param Tbl"=w395) -> ()  [unwired: 8 in, 1 out]
      }
      event "Execute Command": Value Change {
        # "Started one, Unique ID holds\nresponse"
        n257 = event-data() -> ()  [unwired: 1 in, 1 out]
        n258 = property on="Command Selection" class="MCListbox (strict)"() -> ("ItemNames"=w407:string[][])  [unwired: 2 in, 2 out]
        n259 = Index Array(array=w407, index (row)="Command Selection", index (col)=0) -> (element=w405:string)
        n260 = call <vilib>:"Invoke Commands.vi"("Command Params"="Command Params", "Function Name"=w405) -> ("Params"=w401:u8, "Started"=w400:bool)  [unwired: 7 in, 1 out]
        n261 = Array Subset(array="Command Params", length (row)=w401) -> (w402:string[][])  [unwired: 3 in]
        n262 = Select(t="Executing" ("Cmd Status"), s=w400, f="" ("Cmd Status")) -> (s? t:f=→"Cmd Status":string)
      }
      event "Command Selection": Double Click {
        n263 = event-data() -> ("Row"=w415:i32)  [unwired: 1 in]
        n264 = property on="Command Selection" class="MCListbox (strict)"() -> ("ItemNames"=w418:string[][])  [unwired: 2 in, 2 out]
        n265 = local read "Command Params"() -> (w414:string[][])
        n266 = Index Array(array=w418, index (row)=w415, index (col)=0) -> (element=w416:string)
        n267 = call <vilib>:"Invoke Commands.vi"("Command Params"=w414, "Function Name"=w416) -> ("Params"=w413:u8, "Started"=w408:bool)  [unwired: 7 in, 1 out]
        n268 = Array Subset(array=w414, length (row)=w413) -> (w412:string[][])  [unwired: 3 in]
        n269 = Select(t="Executing" ("Cmd Status"), s=w408, f="" ("Cmd Status")) -> (s? t:f=w409:string)
        n270 = local write "Cmd Status"(w409) -> ()
      }
      event "CheckList": Double Click {
        # "Shift clears all"
        # "Update symbols on the listbox"
        n271 = event-data() -> ("PlatMods.Shift"=w420:bool, "Row"=w422:i32)  [unwired: 1 in]
        n272 = case shown="True" w420 {
          tunnel: w422 -> [w426 _]
          tunnel: 1 -> [w425 _]
          frame False {
            n273 = property on="CheckList" class="LstBox (strict)"() -> ("Item Symbols"=w424:i32[])  [unwired: 2 in, 2 out]
            n274 = Replace Array Subset(array=w424, new element=w425, index=w426) -> (w423:i32[])
            n275 = property on="CheckList" class="LstBox (strict)"("Item Symbols"=w423) -> ()  [unwired: 2 in, 2 out]
          }
          frame True {
            w427 = 0 ("Top Row")
            n276 = property on="CheckList" class="LstBox (strict)"() -> ("Number of Rows"=w429:u32)  [unwired: 2 in, 2 out]
            n277 = Initialize Array(0, w429) -> (w428:i32[])
            n278 = property on="CheckList" class="LstBox (strict)"("Top Row"=w427, "Value"=w427, "Item Symbols"=w428) -> ()  [unwired: 2 in, 2 out]
          }
        }
      }
      event "CheckList": Key Down {
        # "Update symbols on the listbox\nLeft and right keys check and uncheck"
        n279 = event-data() -> ("VKey"=w433:T20)  [unwired: 1 in]
        n280 = case shown="\"Left\", \"Right\"" w433 {
          selector: w433 -> [w438 _]
          tunnel: eventvkey."Left" ("VKey") -> [w436 _]
          frame "Left", "Right" {
            n281 = Equal?(x=w436, y=w438) -> (x = y?=w437:bool)
            n282 = Select(t=0, s=w437, f=1) -> (s? t:f=w439:i32)
            n283 = property on="CheckList" class="LstBox (strict)"() -> ("Item Symbols"=w442:i32[])  [unwired: 2 in, 2 out]
            n284 = Replace Array Subset(array=w442, new element=w439, index="CheckList") -> (w441:i32[])
            n285 = property on="CheckList" class="LstBox (strict)"("Item Symbols"=w441) -> ()  [unwired: 2 in, 2 out]
          }
          frame Default {
          }
        }
      }
      event "Motor.Enable": Value Change {
        # "When the test mode otor enable helper is set, update that\ntree row item's value"
        n286 = event-data() -> ("NewVal"=w448:bool)  [unwired: 1 in]
        n287 = Unbundle("Motor") -> ("Value"=w447:dbl)  [unwired: 1 out]
        n288 = Select(t=w447, s=w448, f=0.0) -> (s? t:f=w445:dbl)
        n289 = call <vilib>:"NT Write Number.vi"("Numeric"=w445, "Name"=w444) -> ()  [unwired: 9 in, 1 out]
      }
      event "Test Slider": Value Change {
        # "When the test mode slider helper is set, update that\ntree row item's value"
        n290 = event-data() -> ("NewVal"=w451:dbl)  [unwired: 1 in]
        n291 = call <vilib>:"NT Write Number.vi"("Numeric"=w451, "Name"=w452) -> ()  [unwired: 9 in, 1 out]
      }
      event "On/Off": Value Change {
        # "When the test mode on/off helper value is set, update that\ntree row item's value"
        n292 = event-data() -> ("NewVal"=w456:bool)  [unwired: 1 in]
        n293 = Boolean To (0,1)(Boolean=w456) -> (0, 1=w455:i16)
        n294 = call <vilib>:"NT Write Number.vi"("Numeric"=w455, "Name"=w454) -> ()  [unwired: 9 in, 1 out]
      }
      event "Rev/Fwd": Value Change {
        # "When the test mode helper value for relays is set, update that\ntree row item's value"
        n295 = event-data() -> ("NewVal.Forward"=w464:bool, "NewVal.Reverse"=w463:bool)  [unwired: 1 in]
        n296 = Boolean To (0,1)(Boolean=w464) -> (0, 1=w460:i16)
        n297 = Boolean To (0,1)(Boolean=w463) -> (0, 1=w462:i16)
        n298 = Negate(x=w462) -> (-x=w461:i16)
        n299 = Add(x=w460, y=w461) -> (x+y=w459:i16)
        n300 = call <vilib>:"NT Write Number.vi"("Numeric"=w459, "Name"=w458) -> ()  [unwired: 9 in, 1 out]
      }
      event "Test Ring": Value Change {
        # "When a test mode helper value is selected from the ring,\nset the tree item's variable to the string value"
        n301 = event-data() -> ("NewVal"=w468:u16)  [unwired: 1 in]
        n302 = property on="Test Ring" class="Ring (strict)"() -> ("Strings []"=w469:string[])  [unwired: 2 in, 2 out]
        n303 = Index Array(array=w469, index=w468) -> (element=w467:string)
        n304 = call <vilib>:"NT Write String.vi"("String"=w467, "Name"=w466) -> ()  [unwired: 9 in, 1 out]
      }
      event "Rec Mode": Value Change {
        # "Update globals for recording mode and path to read log from.\nClear when logging and let NetworkTables set path for vision to\nuse."
        n305 = event-data() -> ("NewVal"=w480:enum32{"Stop", "Record", "Playback"})  [unwired: 1 in]
        n306 = global write "WPI_DashboardLogging Global.vi" "Logging Filename"(path "") -> ()
        n307 = global write "WPI_DashboardLogging Global.vi" "Recording"(w480) -> ()
        n308 = case shown="\"Playback\"" w480 {
          tunnel: w479 -> [_ w482 w491]
          tunnel: [_ _ w490] -> w477
          tunnel: [_ _ w489] -> _
          tunnel: w475 -> [_ _ w487]
          tunnel: cluster{i32, i32} {-250, 170} -> [_ _ w486]
          tunnel: [_ _ T21 {"Image Size"=TRUE, "Image Type"=TRUE, "Pixel Value"=TRUE, "ROI Information"=TRUE, "Zoom Factor"=FALSE} ("Image Information Shown:All Elements")] -> w470
          tunnel: [_ _ TRUE ("Zoom Factor")] -> w471
          tunnel: w473 -> [_ _ w483]
          frame Default {
          }
          frame "Stop", "Record" {
            # "Place Window too"
            n309 = invoke class="VI" method="FP.Close"(reference=w482) -> (reference out=w481:refnum<vi>)  [unwired: 2 in, 2 out]
            n310 = invoke class="VI" method="Abort VI"(reference=w481) -> ()  [unwired: 2 in, 3 out]
          }
          frame "Playback" {
            n311 = call "Open Playback Panel.vi"("Offset"=w486, "DB VI Ref"=w487, "Playback in"=w491) -> ("Playback out"=w488:refnum<vi>)  [unwired: 8 in]
            n312 = register-events(w488, w483) -> (reference out=w490:refnum<event-registration>, error out=w489:errorcluster)  [unwired: 2 in]
          }
        }
        n313 = property on="Camera Image Right" class="ImageControl"("Image Information Shown"=w470, "Image Information Visible"=w471) -> ()  [unwired: 2 in, 2 out]
        n314 = property on="Camera Image" class="ImageControl"("Image Information Shown"=w470, "Image Information Visible"=w471) -> ()  [unwired: 2 in, 2 out]
        n315 = call <vilib>:"WPI_DashboardNT Log FieldName Cache.vi"("Operation"=enum16{"Lookup/Add", "Index", "Clear"}."Clear") -> ()  [unwired: 8 in, 3 out]
      }
      event Panel Close {
        w493 = enum32{"Stop", "Record", "Playback"}."Stop" ("Rec Mode")
        # "Playback window has been closed, abort"
        n316 = event-data() -> ()  [unwired: 1 in, 4 out]
        n317 = local write "Rec Mode"(w493) -> ()
        n318 = global write "WPI_DashboardLogging Global.vi" "Recording"(w493) -> ()
      }
      event Panel Close {
        # "Abort playback window and ourself"
        n319 = event-data() -> ()  [unwired: 1 in, 4 out]
        n320 = invoke class="VI" method="FP.Close"(reference=w497) -> (reference out=w496:refnum<vi>)  [unwired: 2 in, 2 out]
        n321 = invoke class="VI" method="Abort VI"(reference=w496) -> (error out=w495:errorcluster)  [unwired: 2 in, 2 out]
        n322 = invoke class="VI" method="Abort VI"(error in=w495) -> ()  [unwired: 2 in, 3 out]
      }
      event User Event {
        n323 = event-data() -> ("IDs"=w504:cluster{"RPC field ID":u16, "Unique ID":u16}, "String"=w503:string)  [unwired: 1 in]
        n324 = Bundle("IDs"=w504, "String"=w503) -> (w502:T9)  [unwired: 1 in]
        n325 = call <vilib>:"Retrieve RPC Response.vi"("RPC Response"=w502) -> ("Output"=w500:string[][])  [unwired: 10 in]
        n326 = Build Array (concatenate)(w498, w500) -> (w499:string[][])
        n327 = local write "Command Params"(w499) -> ()
        n328 = local write "Cmd Status"("" ("Cmd Status")) -> ()
      }
      event "Tree": Double Click {
        n329 = event-data() -> ("PlatMods"=w510:T24, "Tag"=w507:string)  [unwired: 1 in]
        n330 = Unbundle(w510) -> ("Shift"=w509:bool)  [unwired: 4 out]
        n331 = String Subset(string=w507, length (rest)=1 ("length (rest)")) -> (substring=w506:string)  [unwired: 1 in]
        n332 = Not(x=w509) -> (.not. x?=w508:bool)
        n333 = case shown="\"/\"" w506 {
          tunnel: w507 -> [_ w513]
          tunnel: w508 -> [_ w512]
          frame Default {
          }
          frame "/" {
            n334 = call <vilib>:"NT Update Persistence.vi"("Persistence"=w512, "Name"=w513) -> ()  [unwired: 9 in, 1 out]
          }
        }
      }
    }
  }
  n335 = property on="On/Off" class="Bool (strict)"("Visible"=w35) -> ()  [unwired: 2 in, 2 out]
  n336 = property on="Motor" class="Clust (strict)"("Visible"=w35) -> ()  [unwired: 2 in, 2 out]
  n337 = property on="Progress" class="Clust (strict)"("Visible"=w35) -> ()  [unwired: 2 in, 2 out]
  n338 = property on="Test Ring" class="Ring (strict)"("Visible"=w35) -> ()  [unwired: 2 in, 2 out]
  n339 = property on="Rev/Fwd" class="Clust (strict)"("Visible"=w35) -> ()  [unwired: 2 in, 2 out]
  n340 = local write "Command Selection"(u16 0 ("milliseconds to wait")) -> ()
  n341 = while {
    tunnel: u16 1741 ("timeout ms (25000)") -> [w515]
    stop <- FALSE stop-if-true
    n342 = TCP Create Listener(10:w515) -> (0:w514:errorcluster, 3:w516:refnum<k5>)  [unwired: 4 in, 1 out]
    n343 = case shown="No Error" w514 {
      selector: w514 -> [w518 _]
      tunnel: w516 -> [w519 _]
      frame No Error {
        n344 = while {
          tunnel: w519 -> [w522]
          tunnel: w518 -> [w521]
          stop <- FALSE stop-if-true
          n345 = TCP Wait On Listener(8:w521, 11:w522) -> (0:w523:errorcluster, 4:w524:refnum<k5>)  [unwired: 2 in, 3 out]
          n346 = local write "TCP"(w524) -> ()
          n347 = case shown="No Error" w523 {
            frame No Error {
            }
            frame Error {
              n348 = Wait (ms)(milliseconds to wait=u32 1000) -> ()  [unwired: 1 out]
            }
          }
        }
      }
      frame Error {
        n349 = Wait (ms)(milliseconds to wait=u32 1000) -> ()  [unwired: 1 out]
      }
    }
  }
  n350 = local write "Command Params"(string[][] [] ("Command Params")) -> ()
  n351 = global write "WPI_DashboardLogging Global.vi" "Recording"(w58) -> ()
  n352 = local write "Rec Mode"(w58) -> ()
  n353 = call <vilib>:"NT Write String.vi"("Name"="Auto Selector") -> ()  [unwired: 10 in, 1 out]
